vi "Returning Values By Reference Array Of Integers Complete.vi"() -> ()   [LabVIEW 2009, in "LabVIEWWrapper_PassingDataSampleDLL.lvlib"]
uses:
  LabVIEWWrapper_PassingDataSampleDLL.lvlib
panel:
  out "Value":i32[](array[numeric])
  in  "x":i32[](array[numeric])=array[4097 elements]
  in  "length":i32
  in  "error in (no error)":errorcluster
  out "newLength out":i32
  out "newArray out":i32
  out "error out":errorcluster
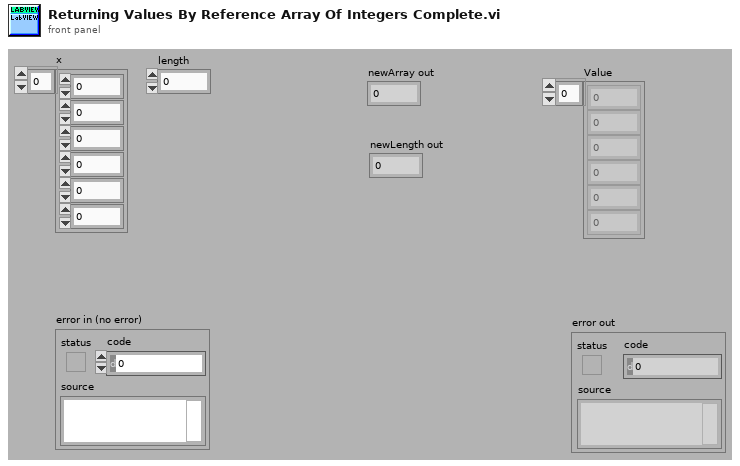
[diagram p1: front panel]
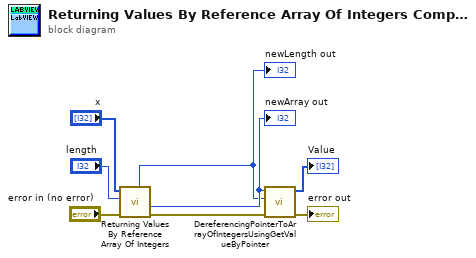
[diagram p0: block diagram]
diagram:
  n1 = call "Returning Values By Reference Array Of Integers.vi"("error in (no error)"="error in (no error)", "length"="length", "x"="x") -> ("error out"=w5:errorcluster, "newArray out"=w3:i32, "newLength out"=w2:i32)  [unwired: 5 in, 1 out]
  "newArray out" <- w3
  "newLength out" <- w2
  n2 = call "DereferencingPointerToArrayOfIntegersUsingGetValueByPointer.vi"("error in (no error)"=w5, "Length"=w2, "Address (Pointer)"=w3) -> ("error out"=→"error out":errorcluster, "Value"=→"Value":i32[])  [unwired: 7 in]
